vi "VisualInspectionEBAY.vi"(8 "error in (no error)":errorcluster, 11 "TableRef":refnum<vi>) -> (0 "error out":errorcluster, 2 "VisualInspectionResult":bool)   [LabVIEW 2017]
panel:
  in  "13":dbl
  in  "17.1":dbl
  in  "16.3":dbl
  in  "16.2":dbl
  in  "16.1":dbl
  in  "15.2":dbl
  in  "15.1":dbl
  in  "14.1":dbl
  in  "12.4":dbl
  in  "12.3":dbl
  in  "12.2":dbl
  in  "12.1":dbl
  in  "11.1":dbl
  in  "18":bool
  in  "10.2":bool
  in  "10.1":bool
  in  "Cancel Button":bool
  in  "OK Button":bool
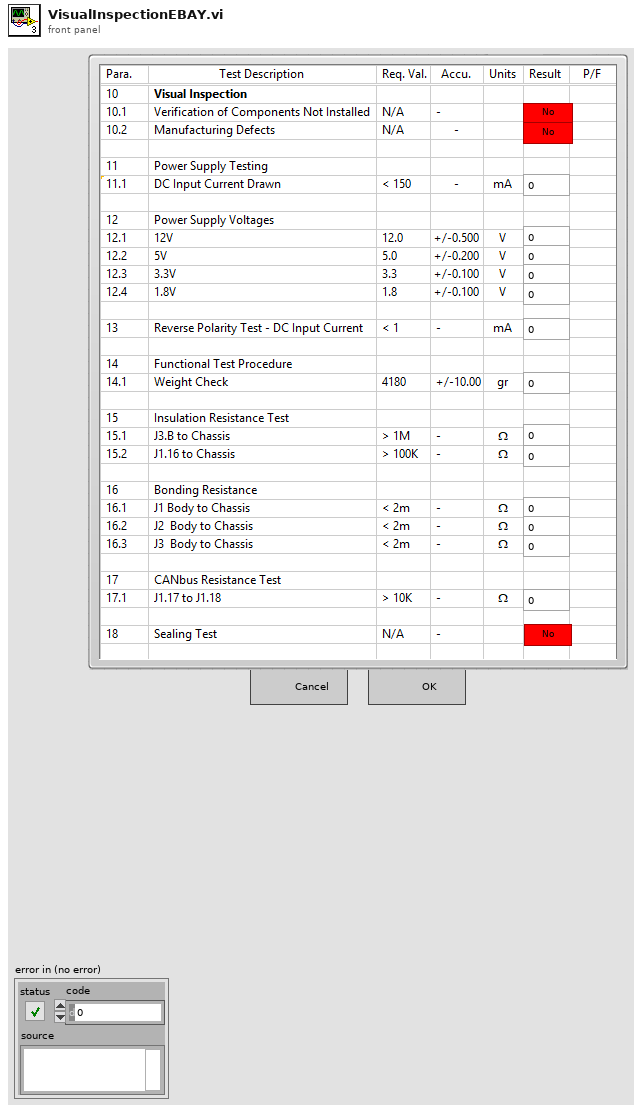
[diagram p1: front panel]
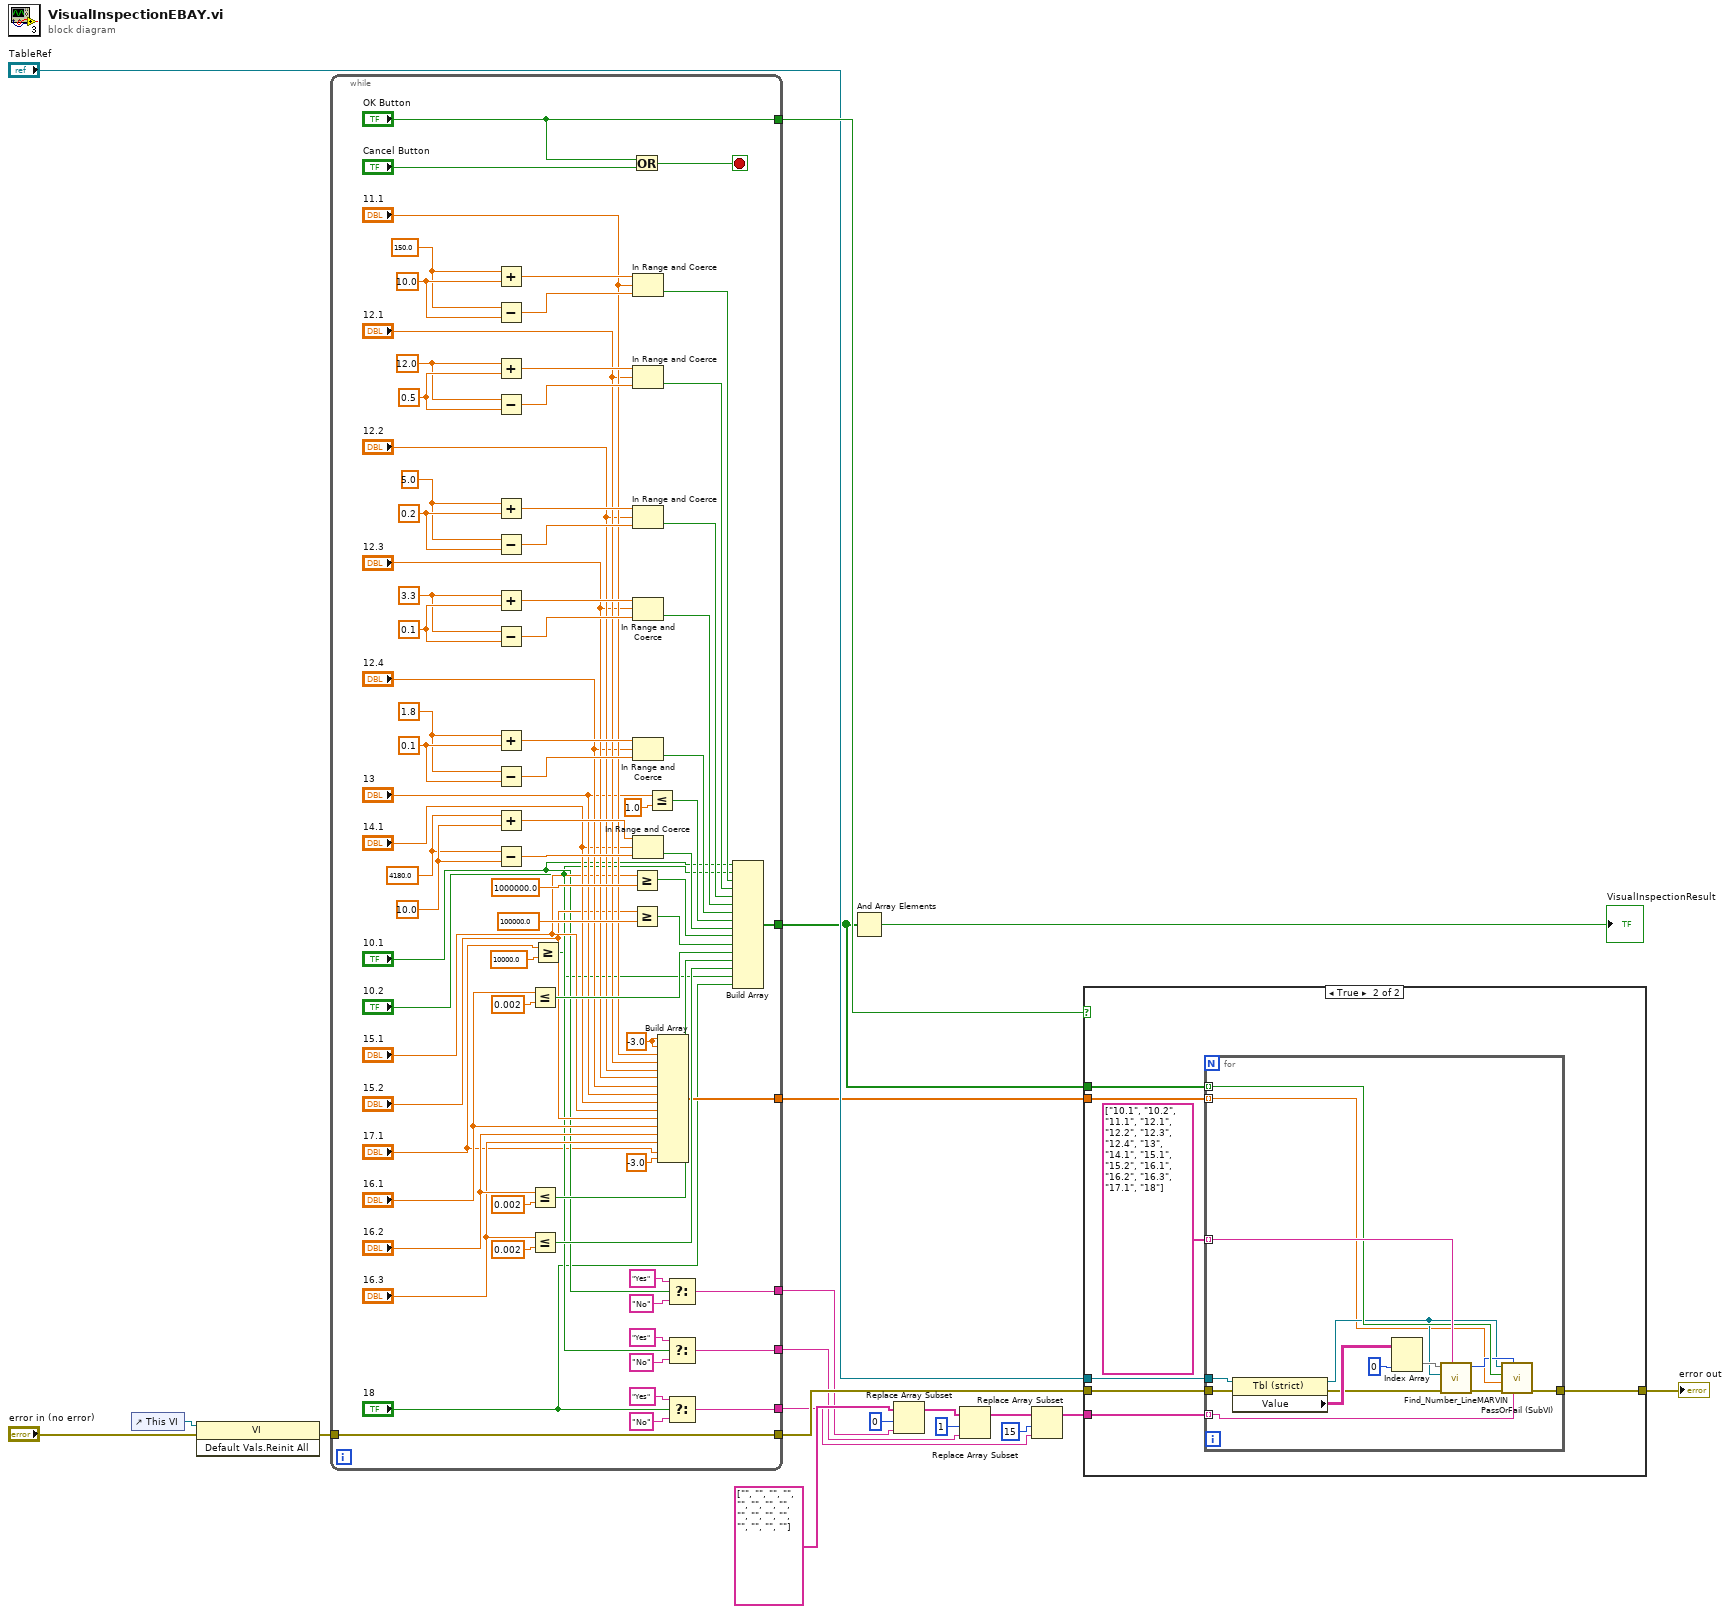
[diagram p0: block diagram]
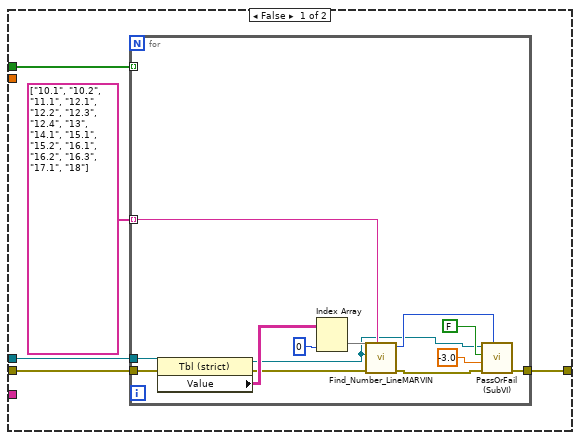
[diagram p2: hidden frame]
diagram:
  n1 = control-ref of="This VI"() -> (w16:refnum<vi>)
  n2 = invoke class="VI" method="Default Vals.Reinit All"(reference=w16, error in="error in (no error)") -> (error out=w20:errorcluster)  [unwired: 1 in, 2 out]
  n3 = while {
    tunnel: w20 -> [w93]
    tunnel: [w95] -> w13
    tunnel: ["OK Button"] -> w19
    tunnel: [w93] -> w18
    tunnel: [w48] -> w11
    tunnel: [w27] -> w4
    tunnel: [w26] -> w3
    tunnel: [w25] -> w2
    stop <- w96 stop-if-true
    w49 = -3.0 ("element")
    w72 = 0.5 ("y")
    w74 = 0.2 ("y")
    w76 = 0.1 ("y")
    w78 = 0.1 ("y")
    w80 = 10.0 ("y")
    w70 = 10.0 ("y")
    w79 = 4180.0 ("y")
    w77 = 1.8 ("y")
    w75 = 3.3 ("y")
    w73 = 5.0 ("y")
    w71 = 12.0 ("y")
    w69 = 150.0 ("y")
    n4 = Add(x=w69, y=w70) -> (x+y=w81:dbl)
    n5 = Subtract(x=w69, y=w70) -> (x-y=w82:dbl)
    n6 = Add(x=w71, y=w72) -> (x+y=w83:dbl)
    n7 = Subtract(x=w71, y=w72) -> (x-y=w84:dbl)
    n8 = Add(x=w73, y=w74) -> (x+y=w85:dbl)
    n9 = Subtract(x=w73, y=w74) -> (x-y=w86:dbl)
    n10 = Add(x=w75, y=w76) -> (x+y=w87:dbl)
    n11 = Subtract(x=w75, y=w76) -> (x-y=w88:dbl)
    n12 = Add(x=w77, y=w78) -> (x+y=w89:dbl)
    n13 = Subtract(x=w77, y=w78) -> (x-y=w90:dbl)
    n14 = Add(x=w79, y=w80) -> (x+y=w91:dbl)
    n15 = Subtract(x=w79, y=w80) -> (x-y=w92:dbl)
    n16 = Less Or Equal?(x="16.1", y=0.002) -> (x <= y?=w52:bool)
    n17 = Less Or Equal?(x="16.2", y=0.002) -> (x <= y?=w51:bool)
    n18 = Less Or Equal?(x="16.3", y=0.002) -> (x <= y?=w50:bool)
    n19 = Greater Or Equal?(x="17.1", y=10000.0) -> (x >= y?=w23:bool)
    n20 = Or(x="OK Button", y="Cancel Button") -> (x .or. y?=w96:bool)
    n21 = Greater Or Equal?(x="15.1", y=1000000.0) -> (x >= y?=w54:bool)
    n22 = Greater Or Equal?(x="15.2", y=100000.0) -> (x >= y?=w53:bool)
    n23 = In Range and Coerce(upper limit=w81, x="11.1", lower limit=w82) -> (In Range?=w61:bool)  [unwired: 1 out]
    n24 = In Range and Coerce(upper limit=w83, x="12.1", lower limit=w84) -> (In Range?=w60:bool)  [unwired: 1 out]
    n25 = In Range and Coerce(upper limit=w85, x="12.2", lower limit=w86) -> (In Range?=w59:bool)  [unwired: 1 out]
    n26 = In Range and Coerce(upper limit=w87, x="12.3", lower limit=w88) -> (In Range?=w58:bool)  [unwired: 1 out]
    n27 = In Range and Coerce(upper limit=w89, x="12.4", lower limit=w90) -> (In Range?=w57:bool)  [unwired: 1 out]
    n28 = In Range and Coerce(upper limit=w91, x="14.1", lower limit=w92) -> (In Range?=w55:bool)  [unwired: 1 out]
    n29 = Less Or Equal?(x="13", y=1.0) -> (x <= y?=w56:bool)
    n30 = Build Array(w49, w49, "11.1", "12.1", "12.2", "12.3", "12.4", "13", "14.1", "15.1", "15.2", "16.1", "16.2", "16.3", "17.1", -3.0 ("element")) -> (w48:dbl[])
    n31 = Select(t="Yes", s="10.1", f="No") -> (s? t:f=w25:string)
    n32 = Select(t="Yes", s="10.2", f="No") -> (s? t:f=w26:string)
    n33 = Select(t="Yes", s="18", f="No") -> (s? t:f=w27:string)
    n34 = Build Array("10.1", "10.2", w61, w60, w59, w58, w57, w56, w55, w54, w53, w52, w51, w50, w23, "18") -> (w95:bool[])
  }
  n35 = And Array Elements(Boolean array=w13) -> (logical AND=→"VisualInspectionResult":bool)
  n36 = Replace Array Subset(array=string[] ["", "", "", "", "", "", "", "", "", "", "", "", "", "", "", ""], new element=w2, index=0) -> (w9:string[])
  n37 = Replace Array Subset(array=w9, new element=w3, index=1) -> (w8:string[])
  n38 = Replace Array Subset(array=w8, new element=w4, index=15) -> (w1:string[])
  n39 = case shown="True" w19 {
    tunnel: w13 -> [w102 w122]
    tunnel: w18 -> [w101 w121]
    tunnel: [w100 w120] -> w14
    tunnel: "TableRef" -> [w99 w119]
    tunnel: w11 -> [_ w117]
    tunnel: w1 -> [_ w116]
    frame False {
      n40 = for {
        tunnel: string[] ["10.1", "10.2", "11.1", "12.1", "12.2", "12.3", "12.4", "13", "14.1", "15.1", "15.2", "16.1", "16.2", "16.3", "17.1", "18"] ("Array 4") -> [w111] mode=indexing
        tunnel: w102 -> [_] mode=indexing
        tunnel: w101 -> [w108]
        tunnel: [w107] -> w100
        tunnel: w99 -> [w106]
        n41 = property class="Tbl (strict)"(reference=w106, error in=w108) -> (reference out=w104:refnum<vi>, error out=w112:errorcluster, "Value"=w115:string[][])
        n42 = Index Array(array=w115, index (col)=0 ("disabled index (col)")) -> (element=w113:string[])  [unwired: 1 in]
        n43 = call "Find_Number_LineMARVIN.vi"("Test Paragraph"=w111, "error in"=w112, "TableIn"=w104, "Row Headers[]"=w113) -> ("error out"=w110:errorcluster, "Line number"=w109:i32)  [unwired: 1 in, 2 out]
        n44 = call "PassOrFail (SubVI).vi"("index (row)"=w109, "error in (no error)"=w110, "Data in"=-3.0, "Pass?Fail"=FALSE ("Boolean"), "Table in"=w104) -> ("error out"=w107:errorcluster)  [unwired: 6 in]
      }
    }
    frame True {
      n45 = for {
        tunnel: string[] ["10.1", "10.2", "11.1", "12.1", "12.2", "12.3", "12.4", "13", "14.1", "15.1", "15.2", "16.1", "16.2", "16.3", "17.1", "18"] ("Array 4") -> [w132] mode=indexing
        tunnel: w122 -> [w130] mode=indexing
        tunnel: w121 -> [w128]
        tunnel: [w127] -> w120
        tunnel: w119 -> [w126]
        tunnel: w117 -> [w124] mode=indexing
        tunnel: w116 -> [w123] mode=indexing
        n46 = property class="Tbl (strict)"(reference=w126, error in=w128) -> (reference out=w125:refnum<vi>, error out=w133:errorcluster, "Value"=w136:string[][])
        n47 = Index Array(array=w136, index (col)=0 ("disabled index (col)")) -> (element=w134:string[])  [unwired: 1 in]
        n48 = call "Find_Number_LineMARVIN.vi"("Test Paragraph"=w132, "error in"=w133, "TableIn"=w125, "Row Headers[]"=w134) -> ("error out"=w131:errorcluster, "Line number"=w129:i32)  [unwired: 1 in, 2 out]
        n49 = call "PassOrFail (SubVI).vi"("String Res"=w123, "index (row)"=w129, "error in (no error)"=w131, "Data in"=w124, "Pass?Fail"=w130, "Table in"=w125) -> ("error out"=w127:errorcluster)  [unwired: 5 in]
      }
    }
  }
  "error out" <- w14
